vi "Configure Time Unit.vi"(0 "VISA resource name":refnum<visa-resource-name>, 5 "Time Unit (Seconds)":enum16{"Seconds", "Minutes", "Hours"}(ring), 11 "error in (no error)":errorcluster) -> (4 "VISA resource name out":refnum<visa-resource-name>, 15 "error out":errorcluster)   [LabVIEW 2016, in "APT 300XAC Series.lvlib"]
doc: "Sets the <B>time unit</B> to the power source instrument.\n\n<B>Range</B>\n[Seconds, Minutes, Hour]\n\nNot supported in manual mode.\n\nProgram mode: this is a system parameter.\n\n\nThe timer unit parameter determines the time increment that will be used for testing when the source is in the program mode. The operator can select between SECOND/MINUTE/HOUR."
uses:
  APT 300XAC Series.lvlib
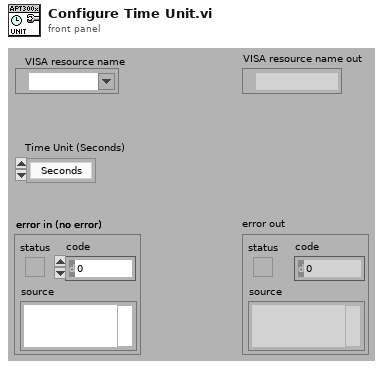
[diagram p1: front panel]
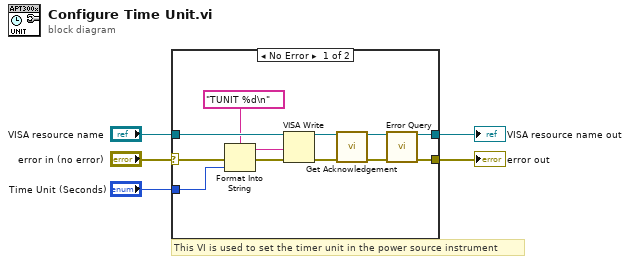
[diagram p0: block diagram]
diagram:
  # "This VI is used to set the timer unit in the power source instrument"
  n1 = case shown="No Error" "error in (no error)" {
    selector: "error in (no error)" -> [w13 w19]
    tunnel: "VISA resource name" -> [w17 w18]
    tunnel: [w15 w18] -> w4
    tunnel: [w14 w19] -> w3
    tunnel: "Time Unit (Seconds)" -> [w11 _]
    frame No Error {
      n2 = Format Into String(format string="TUNIT %d\n" ("Command"), error in=w13, w11) -> (resulting string=w16:string, error out=w12:errorcluster)  [unwired: 1 in]
      n3 = VISA Write(VISA resource name=w17, write buffer=w16, error in (no error)=w12) -> (VISA resource name out=w6:refnum<visa-resource-name>, error out=w7:errorcluster)  [unwired: 1 out]
      n4 = call "Get Acknowledgement.vi"("VISA resource name"=w6, "error in (no error)"=w7) -> ("VISA resource name out"=w9:refnum<visa-resource-name>, "error out"=w8:errorcluster)  [unwired: 12 in]
      n5 = call "Error Query.vi"("VISA resource name"=w9, "error in (no error)"=w8) -> ("VISA resource name out"=w15:refnum<visa-resource-name>, "error out"=w14:errorcluster)  [unwired: 10 in, 2 out]
    }
    frame Error {
    }
  }
  "error out" <- w3
  "VISA resource name out" <- w4
